vi "Server_Search Data.vi"(8 "error in":errorcluster, 11 "connection ID":refnum<k5>) -> (0 "error out":errorcluster)   [LabVIEW 2018, in "Cloud Server.lvlib"]
uses:
  Cloud Server.lvlib
  Data Def/Server_Connection Manager Method.ctl
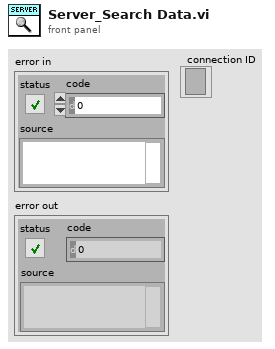
[diagram p1: front panel]
types:
  T1 = typedef "Cloud Server.lvlib/Server_Connection Manager Method.ctl" = enum16{"Initialize", "Add", "Get", "Set Properties", "Get Properties", "Close", "Release"}
  T2 = typedef "Cloud Server.lvlib/Server_Main Data.ctl" = cluster{"Main VI Ref.":refnum<vi>, "Listener ID":refnum<k5>, "Meta data":T3[], "Main Queue":T5, "User Picture":T6}
  T3 = typedef "stm_MetaElement.ctl" = cluster{"Name":T4}
  T4 = typedef "stm_MetaDataElement.ctl" = string
  T5 = typedef "Cloud Server.lvlib/Server_Main Queue.ctl" = cluster{"Server Write Queue":refnum<queue>, "Main Loop Queue":refnum<queue>}
  T6 = typedef "IMAQ Image.ctl" = refnum<image>
  T7 = typedef "Cloud Server.lvlib/Server_Connection Properties.ctl" = cluster{"User Data":T8, "Data":waveform(dbl)}
  T8 = typedef "User Data.ctl" = cluster{"Name":string, "Email":string, "Phone Number":string, "User Picture":u32[][], "Last Login Time":timestamp}
  T9 = typedef "Data File Format.ctl" = cluster{"Data":waveform(dbl), "Abnormal?":bool, "Measure Time":timestamp, "User Name":string}
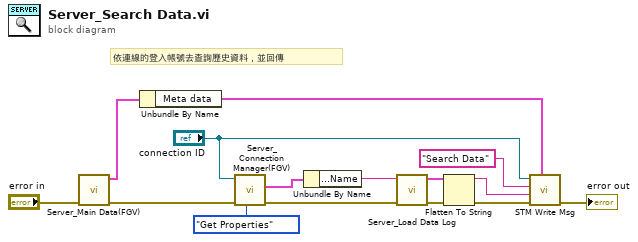
[diagram p0: block diagram]
diagram:
  # "依連線的登入帳號去查詢歷史資料，並回傳"
  n1 = call "Server_Main Data(FGV).vi"("error in"="error in") -> ("error out"=w7:errorcluster, "Main Data Out"=w5:T2)  [unwired: 9 in]
  n2 = Unbundle By Name(w5) -> ("Meta data"=w4:T3[])
  n3 = call "Server_Connection Manager(FGV).vi"("Connection Manager Method(Get)"=Server_Connection_Manager_Method."Get Properties", "error in"=w7, "Connection In"="connection ID") -> ("error out"=w13:errorcluster, "Connection Properties Out"=w14:T7)  [unwired: 4 in, 3 out]
  n4 = Unbundle By Name(w14) -> ("User Data.Name"=w12:string)
  n5 = call "Server_Load Data Log.vi"("error in"=w13, "User Name"=w12) -> ("error out"=w11:errorcluster, "Log Data"=w10:T9[])  [unwired: 8 in]
  n6 = Flatten To String(anything=w10, error in (no error)=w11) -> (data string=w3:string, error out=w9:errorcluster)  [unwired: 2 in, 1 out]
  n7 = call "STM Write Msg.vi"("Meta data"=w4, "error in (no error)"=w9, "Data"=w3, "Name"="Search Data", "connection ID"="connection ID") -> ("error out"=→"error out":errorcluster)  [unwired: 5 in, 1 out]
